vi "Enable.vi"(8 "error in (no error)":errorcluster, 10 "Enable":bool, 11 "DC Motor in":refnum<class "DC Motor.lvclass">) -> (0 "error out":errorcluster, 2 "Message":string, 3 "DC Motor out":refnum<class "DC Motor.lvclass">)   [LabVIEW 2021, in "DC Motor.lvclass"]
uses:
  DC Motor.lvclass
  Actuator/Actuator.lvclass
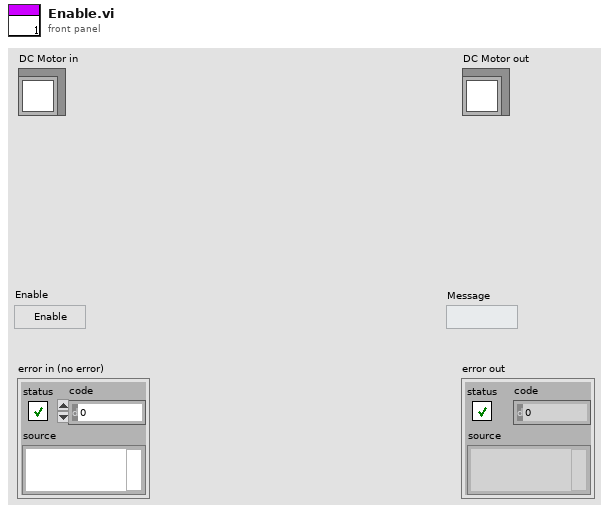
[diagram p1: front panel]
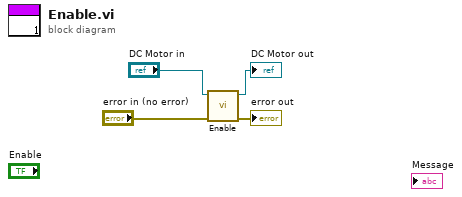
[diagram p0: block diagram]
diagram:
  n1 = call-parent "Enable.vi"("error in (no error)"="error in (no error)", "Actuator in"="DC Motor in") -> ("error out"=→"error out":errorcluster, "Actuator out"=→"DC Motor out":refnum<class "DC Motor.lvclass">)  [unwired: 7 in, 1 out]
